vi "Main Dialog.vi"(11 "Process Path":path) -> ()   [LabVIEW 2020, in "Method Generation.lvlib" / "New Getter Dialog.lvclass"]
uses:
  New Getter Dialog.lvclass
  New Getter Dialog.lvclass/New Getter Dialog.ctl
  Getter Generator/Getter Generator.lvclass
panel:
  in  "Commit":bool
  in  "Cancel":bool
  in  "Data members":i32(listbox)
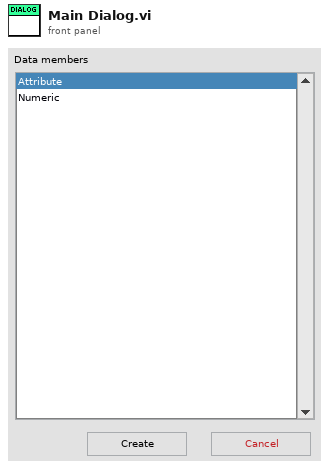
[diagram p1: front panel]
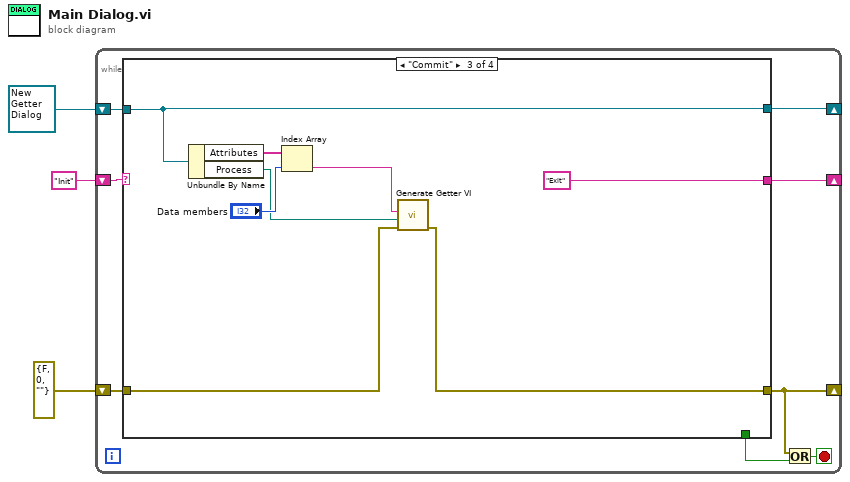
[diagram p0: block diagram]
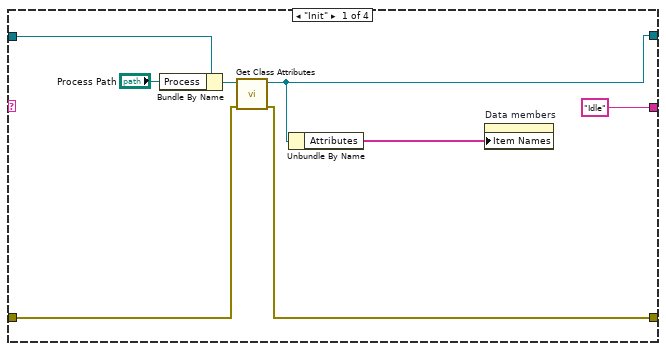
[diagram p2: hidden frame]
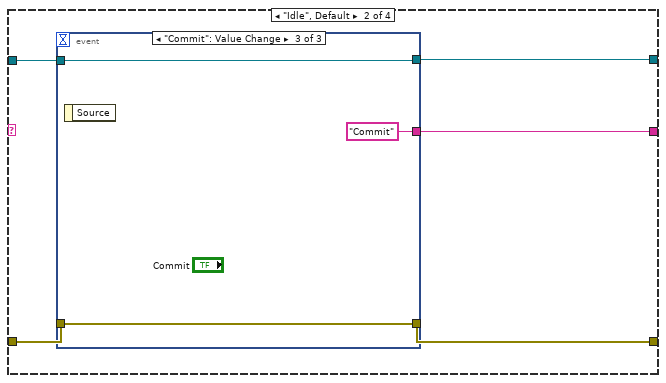
[diagram p3: hidden frame]
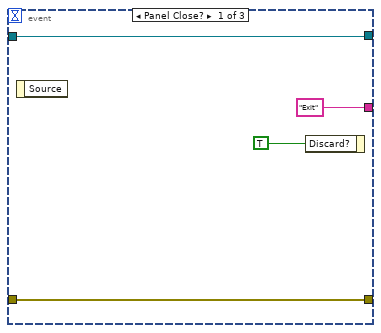
[diagram p4: hidden frame]
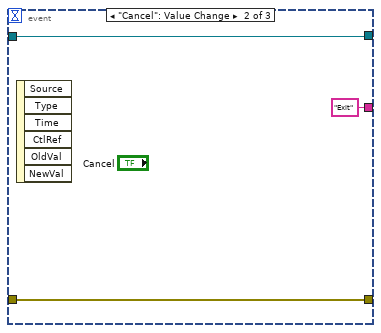
[diagram p5: hidden frame]
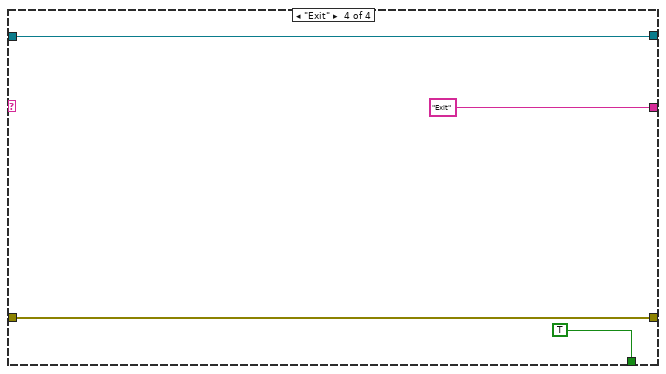
[diagram p6: hidden frame]
diagram:
  n1 = while {
    shift-right: [w8] -> _
    shift-left: refnum<class "New Getter Dialog.lvclass"> refnum ("Method Generation.lvlib:New Getter Dialog.lvclass") -> [w9]
    shift-right: [w4] -> _
    shift-left: errorcluster {"status"=FALSE, "code"=0, "source"=""} ("error in (no error)") -> [w10]
    shift-right: [w7] -> _
    shift-left: "Init" -> [w11]
    stop <- w5 stop-if-true
    n2 = case shown="\"Commit\"" w11 {
      tunnel: [w15 w24 w36 w45] -> w4
      tunnel: w10 -> [w14 w23 w35 w45]
      tunnel: w9 -> [w19 w22 w41 w46]
      tunnel: [w13 w21 w41 w46] -> w8
      tunnel: ["Idle" w20 "Exit" "Exit"] -> w7
      tunnel: [_ _ _ TRUE] -> w6
      frame "Init" {
        n3 = Bundle By Name(cluster=w19, "Process"="Process Path") -> (w16:refnum<class "New Getter Dialog.lvclass">)
        n4 = call "Get Class Attributes.vi"("error in (no error)"=w14, "New Getter Dialog In"=w16) -> ("error out"=w15:errorcluster, "New Getter Dialog Out"=w13:refnum<class "New Getter Dialog.lvclass">)  [unwired: 8 in]
        n5 = Unbundle By Name(w13) -> ("Attributes"=w12:string[])
        n6 = property on="Data members" class="LstBox (strict)"("Item Names"=w12) -> ()  [unwired: 2 in, 2 out]
      }
      frame "Idle", Default {
        n7 = event shown="[2] \"Commit\": Value Change" {
          selector: _ -> [_ _ _]
          dyn-events: _ -> [_ _ _]
          timeout: _ -> [_ _ _]
          tunnel: [w28 w30 w34] -> w24
          tunnel: w23 -> [w28 w30 w34]
          tunnel: w22 -> [w27 w31 w33]
          tunnel: [w27 w31 w33] -> w21
          tunnel: ["Exit" "Exit" "Commit"] -> w20
          event Panel Close? {
            n8 = event-data() -> ()  [unwired: 1 in, 1 out]
            n9 = event-data("Discard?"=TRUE) -> ()  [unwired: 1 in, 1 out]
          }
          event "Cancel": Value Change {
            n10 = event-data() -> ()  [unwired: 1 in, 6 out]
          }
          event "Commit": Value Change {
            n11 = event-data() -> ()  [unwired: 1 in, 1 out]
          }
        }
      }
      frame "Commit" {
        n12 = Unbundle By Name(w41) -> ("Attributes"=w40:string[], "Process"=w37:path)
        n13 = Index Array(array=w40, index="Data members") -> (element=w38:string)
        n14 = call "Generate Getter VI.vi"("error in (no error)"=w35, "class path"=w37, "Attribute Name"=w38) -> ("error out"=w36:errorcluster)  [unwired: 8 in]
      }
      frame "Exit" {
      }
    }
    n15 = Or(x=w4, y=w6) -> (x .or. y?=w5:bool)
  }
